vi "OpenMV.vi"(7 "JPG":refnum<vi>, 10 "queueName":string="PV_script", 11 "Console Reference":refnum<vi>) -> ()   [LabVIEW 2022 SP3]
panel:
  in  "Grab":bool
  in  "Snap":bool
  out "Image":picture
  out "Plots":T1
  in  "start":bool
  # "Camera View"
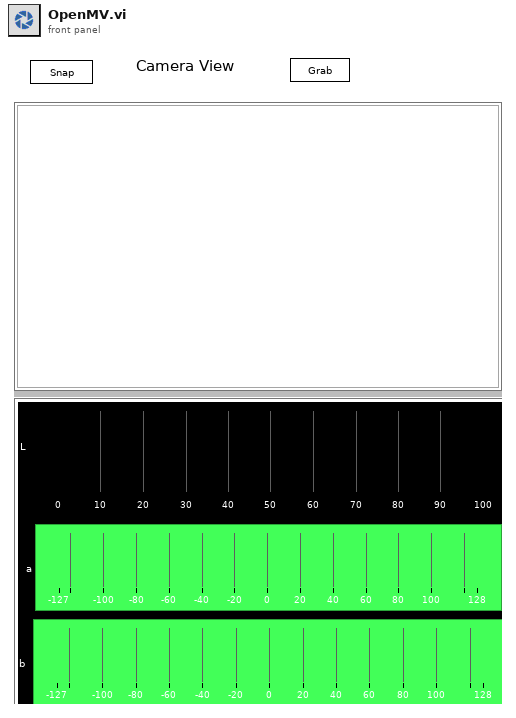
[diagram p1: front panel]
types:
  T1 = cluster{"L":dbl[], "a":cluster{i32, i32, dbl[]}, "b":cluster{i32, i32, dbl[]}}
  T2 = enum16{"read", "write pause", "write port", "write path", "write all"}
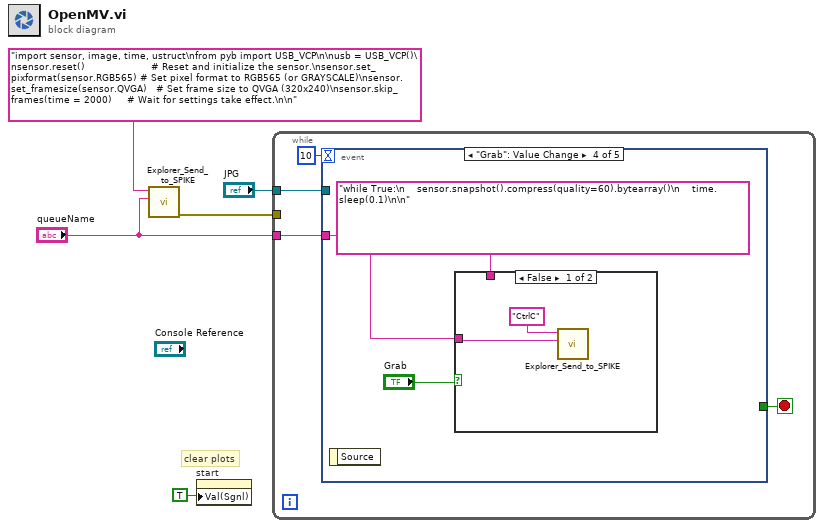
[diagram p0: block diagram]
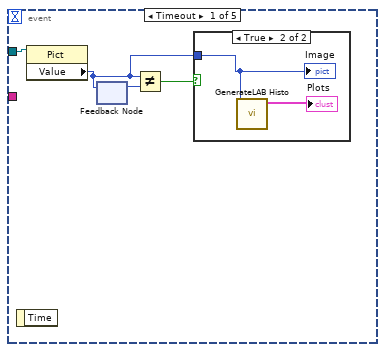
[diagram p2: hidden frame]
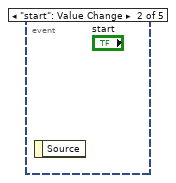
[diagram p4: hidden frame]
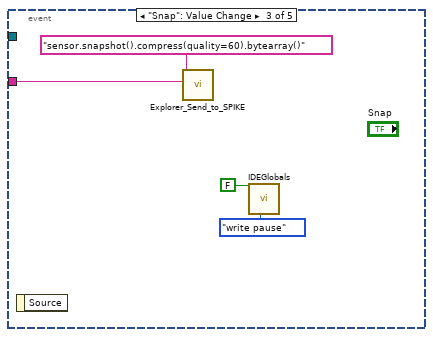
[diagram p5: hidden frame]
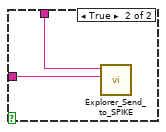
[diagram p6: hidden frame]
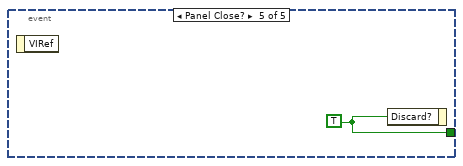
[diagram p7: hidden frame]
diagram:
  # "clear plots"
  n1 = call "Explorer_Send_to_SPIKE.vi"("queueName"="queueName", "python"="import sensor, image, time, ustruct\nfrom pyb import USB_VCP\n\nusb = USB_VCP()\nsensor.reset()                      # Reset and initialize the sensor.\nsensor.set_pixformat(sensor.RGB565) # Set pixel format to RGB565 (or GRAYSCALE)\nsensor.set_framesize(sensor.QVGA)   # Set frame size to QVGA (320x240)\nsensor.skip_frames(time = 2000)     # Wait for settings take effect.\n\n") -> ("error out"=w1:errorcluster)  [unwired: 9 in]
  n2 = property on="start" class="Bool (strict)"("Val(Sgnl)"=TRUE ("Value (Signaling)")) -> ()  [unwired: 2 in, 2 out]
  n3 = while {
    tunnel: "JPG" -> [w7]
    tunnel: "queueName" -> [w6]
    tunnel: w1 -> [_]
    stop <- w8 stop-if-true
    n4 = event shown="[3] \"Grab\": Value Change" {
      selector: _ -> [_ _ _ _ _]
      dyn-events: _ -> [_ _ _ _ _]
      timeout: 10 -> [_ _ _ _ _]
      tunnel: [_ _ _ _ w27] -> w8
      tunnel: w7 -> [w13 _ _ _ _]
      tunnel: w6 -> [_ _ w18 w21 _]
      event Timeout {
        n5 = event-data() -> ()  [unwired: 1 in, 1 out]
        n6 = property on="Property Node" class="Pict"(reference=w13) -> ("Value"=w10:picture)  [unwired: 1 in, 2 out]
        n7 = feedback #1() -> (w12:picture)  [unwired: 1 in]
        n8 = feedback-in #1(w10) -> ()
        n9 = Not Equal?(x=w10, y=w12) -> (x != y?=w11:bool)
        n10 = case shown="True" w11 {
          tunnel: w10 -> [_ w15]
          frame False {
          }
          frame True {
            n11 = call "GenerateLAB Histo.vi"("2D Picture"=w15) -> ("Plots"=→"Plots":T1)  [unwired: 9 in, 1 out]
            "Image" <- w15
          }
        }
      }
      event "start": Value Change {
        n12 = event-data() -> ()  [unwired: 1 in, 1 out]
      }
      event "Snap": Value Change {
        n13 = event-data() -> ()  [unwired: 1 in, 1 out]
        n14 = call "Explorer_Send_to_SPIKE.vi"("queueName"=w18, "python"="sensor.snapshot().compress(quality=60).bytearray()") -> ()  [unwired: 9 in, 1 out]
        n15 = call "IDEGlobals.vi"("task"=T2."write pause", "pause?"=FALSE) -> ()  [unwired: 7 in, 3 out]
      }
      event "Grab": Value Change {
        n16 = event-data() -> ()  [unwired: 1 in, 1 out]
        n17 = case shown="False" "Grab" {
          tunnel: "while True:\n    sensor.snapshot().compress(quality=60).bytearray()\n    time.sleep(0.1)\n\n" ("python") -> [_ w26]
          tunnel: w21 -> [w23 w25]
          frame False {
            n18 = call "Explorer_Send_to_SPIKE.vi"("queueName"=w23, "python"="CtrlC") -> ()  [unwired: 9 in, 1 out]
          }
          frame True {
            n19 = call "Explorer_Send_to_SPIKE.vi"("queueName"=w25, "python"=w26) -> ()  [unwired: 9 in, 1 out]
          }
        }
      }
      event Panel Close? {
        w27 = TRUE ("Discard?")
        n20 = event-data() -> ()  [unwired: 1 in, 1 out]
        n21 = event-data("Discard?"=w27) -> ()  [unwired: 1 in, 1 out]
      }
    }
  }
